vi "Continuous Analog Output Regeneration DAQ.vi"() -> ()   [LabVIEW 2020]
uses:
  <vilib>/DAQmx/write.llb/DAQmx Write (Analog 1D DBL 1Chan NSamp).vi
  <vilib>/DAQmx/create/channels.llb/DAQmx Create Channel (AO-Voltage-Basic).vi
  <vilib>/DAQmx/configure/timing.llb/DAQmx Timing (Sample Clock).vi
  <vilib>/DAQmx/miscellaneous.llb/DAQmx Fill In Error Info.vi
  <resource>/objmgr/daqmx.rc
panel:
  in  "Stop":bool
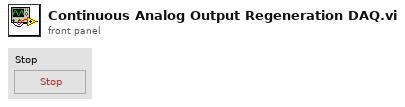
[diagram p1: front panel]
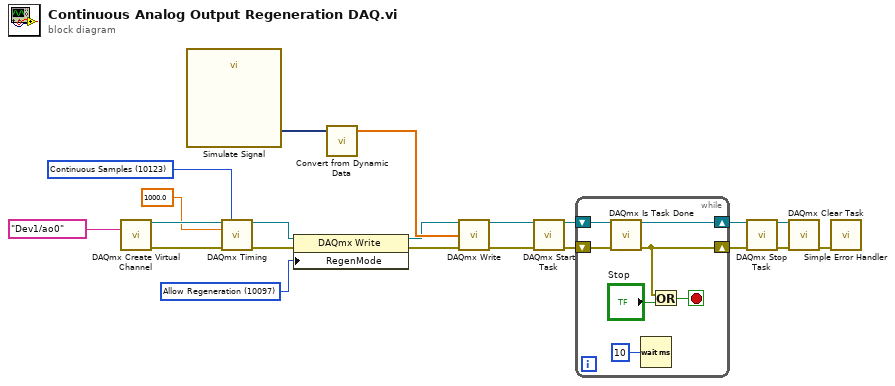
[diagram p0: block diagram]
diagram:
  w1 = 10097 items=["Allow Regeneration"=10097, "Do Not Allow Regeneration"=10158] ("RegenMode")
  w17 = 10123 items=["Finite Samples"=10178, "Continuous Samples"=10123, "Hardware Timed Single Point"=12522] ("sample mode")
  n1 = call-poly <vilib>:"DAQmx Create Virtual Channel.vi"("physical channels"=tag "Dev1/ao0") -> ("task out"=w20:refnum<k21>, "error out"=w19:errorcluster)  [unwired: 13 in]
  n2 = call "Simulate Signal"() -> ("Triangle"=w16:dynamicdata)  [unwired: 14 in, 1 out]
  n3 = call-poly <vilib>:"DAQmx Timing.vi"("task/channels in"=w20, "sample mode"=w17, "rate"=1000.0, "error in"=w19) -> ("task out"=w5:refnum<k21>, "error out"=w4:errorcluster)  [unwired: 10 in]
  n4 = property class="DAQmx Write"(reference=w5, error in=w4, "RegenMode"=w1) -> (reference out=w3:refnum<k21>, error out=w2:errorcluster)
  n5 = call "Convert from Dynamic Data"("Dynamic Data Type"=w16) -> ("Array"=w15:dbl[])  [unwired: 3 in]
  n6 = call-poly <vilib>:"DAQmx Write.vi"("task/channels in"=w3, "data"=w15, "error in"=w2) -> ("task out"=w14:refnum<k21>, "error out"=w13:errorcluster)  [unwired: 10 in, 1 out]
  n7 = call <vilib>:"DAQmx Start Task.vi"("task/channels in"=w14, "error in"=w13) -> ("task out"=w12:refnum<k21>, "error out"=w11:errorcluster)  [unwired: 12 in]
  n8 = while {
    shift-right: [w26] -> w10
    shift-left: w12 -> [w28]
    shift-right: [w24] -> w9
    shift-left: w11 -> [w27]
    stop <- w25 stop-if-true
    n9 = call <vilib>:"DAQmx Is Task Done.vi"("task/channels in"=w28, "error in"=w27) -> ("task out"=w26:refnum<k21>, "error out"=w24:errorcluster)  [unwired: 11 in, 1 out]
    n10 = Wait (ms)(milliseconds to wait=u32 10) -> ()  [unwired: 1 out]
    n11 = Or(x=w24, y="Stop") -> (x .or. y?=w25:bool)
  }
  n12 = call <vilib>:"DAQmx Stop Task.vi"("task/channels in"=w10, "error in"=w9) -> ("task out"=w8:refnum<k21>, "error out"=w7:errorcluster)  [unwired: 12 in]
  n13 = call <vilib>:"DAQmx Clear Task.vi"("task in"=w8, "error in"=w7) -> ("error out"=w6:errorcluster)  [unwired: 13 in]
  n14 = call <vilib>:"Simple Error Handler.vi"("error in (no error)"=w6) -> ()  [unwired: 4 in, 5 out]
